vi "Trio - Disconnect.vi"(9 "TrioData In":T1 {"A Axis Parameters"."VPSPEED" format="%#_4g"; "A Axis Parameters"."AXISSTATUS" format="%#_4g"; "A Axis Parameters"."FE" format="%#_4g"; "A Axis Parameters"."MPOS" format="%#_4g"; "A Axis Parameters"."NTYPE" format="%#_4g"; "A Axis Parameters"."MTYPE" format="%#_4g"; "A Axis Parameters"."RS_LIMIT" format="%#_4g"; "A Axis Parameters"."FS_LIMIT" format="%#_4g"; "A Axis Parameters"."FH_IN" format="%#_4g"; "A Axis Parameters"."DATUM_IN" format="%#_4g"; "A Axis Parameters"."REV_IN" format="%#_4g"; "A Axis Parameters"."FWD_IN" format="%#_4g"; "A Axis Parameters"."REP_DIST" format="%#_4g"; "A Axis Parameters"."SERVO" format="%#_4g"; "A Axis Parameters"."DAC" format="%#_4g"; "A Axis Parameters"."FE_LIMIT" format="%#_4g"; "A Axis Parameters"."JOGSPEED" format="%#_4g"; "A Axis Parameters"."CREEP" format="%#_4g"; "A Axis Parameters"."DECEL" format="%#_4g"; "A Axis Parameters"."ACCEL" format="%#_4g"; "A Axis Parameters"."SPEED" format="%#_4g"; "A Axis Parameters"."UNITS" format="%#_4g"; "A Axis Parameters"."VFF_GAIN" format="%#_4g"; "A Axis Parameters"."0V_GAIN" format="%#_4g"; "A Axis Parameters"."D_GAIN" format="%#_4g"; "A Axis Parameters"."I_GAIN" format="%#_4g"; "A Axis Parameters"."P_GAIN" format="%#_4g"; "A Axis Parameters"."ATYPE" format="%#_4g"; "X Axis Parameters"."VPSPEED" format="%#_4g"; "X Axis Parameters"."AXISSTATUS" format="%#_4g"; "X Axis Parameters"."FE" format="%#_4g"; "X Axis Parameters"."MPOS" format="%#_4g"; "X Axis Parameters"."NTYPE" format="%#_4g"; "X Axis Parameters"."MTYPE" format="%#_4g"; "X Axis Parameters"."RS_LIMIT" format="%#_4g"; "X Axis Parameters"."FS_LIMIT" format="%#_4g"; "X Axis Parameters"."FH_IN" format="%#_4g"; "X Axis Parameters"."DATUM_IN" format="%#_4g"; "X Axis Parameters"."REV_IN" format="%#_4g"; "X Axis Parameters"."FWD_IN" format="%#_4g"; "X Axis Parameters"."REP_DIST" format="%#_4g"; "X Axis Parameters"."SERVO" format="%#_4g"; "X Axis Parameters"."DAC" format="%#_4g"; "X Axis Parameters"."FE_LIMIT" format="%#_4g"; "X Axis Parameters"."JOGSPEED" format="%#_4g"; "X Axis Parameters"."CREEP" format="%#_4g"; "X Axis Parameters"."DECEL" format="%#_4g"; "X Axis Parameters"."ACCEL" format="%#_4g"; "X Axis Parameters"."SPEED" format="%#_4g"; "X Axis Parameters"."UNITS" format="%#_4g"; "X Axis Parameters"."VFF_GAIN" format="%#_4g"; "X Axis Parameters"."0V_GAIN" format="%#_4g"; "X Axis Parameters"."D_GAIN" format="%#_4g"; "X Axis Parameters"."I_GAIN" format="%#_4g"; "X Axis Parameters"."P_GAIN" format="%#_4g"; "X Axis Parameters"."ATYPE" format="%#_4g"}, 10 "error in (no error)":errorcluster, 11 "Trio Reference In":refnum<k7>) -> (1 "TrioData Out":T1 {"A Axis Parameters"."VPSPEED" format="%#_4g"; "A Axis Parameters"."AXISSTATUS" format="%#_4g"; "A Axis Parameters"."FE" format="%#_4g"; "A Axis Parameters"."MPOS" format="%#_4g"; "A Axis Parameters"."NTYPE" format="%#_4g"; "A Axis Parameters"."MTYPE" format="%#_4g"; "A Axis Parameters"."RS_LIMIT" format="%#_4g"; "A Axis Parameters"."FS_LIMIT" format="%#_4g"; "A Axis Parameters"."FH_IN" format="%#_4g"; "A Axis Parameters"."DATUM_IN" format="%#_4g"; "A Axis Parameters"."REV_IN" format="%#_4g"; "A Axis Parameters"."FWD_IN" format="%#_4g"; "A Axis Parameters"."REP_DIST" format="%#_4g"; "A Axis Parameters"."SERVO" format="%#_4g"; "A Axis Parameters"."DAC" format="%#_4g"; "A Axis Parameters"."FE_LIMIT" format="%#_4g"; "A Axis Parameters"."JOGSPEED" format="%#_4g"; "A Axis Parameters"."CREEP" format="%#_4g"; "A Axis Parameters"."DECEL" format="%#_4g"; "A Axis Parameters"."ACCEL" format="%#_4g"; "A Axis Parameters"."SPEED" format="%#_4g"; "A Axis Parameters"."UNITS" format="%#_4g"; "A Axis Parameters"."VFF_GAIN" format="%#_4g"; "A Axis Parameters"."0V_GAIN" format="%#_4g"; "A Axis Parameters"."D_GAIN" format="%#_4g"; "A Axis Parameters"."I_GAIN" format="%#_4g"; "A Axis Parameters"."P_GAIN" format="%#_4g"; "A Axis Parameters"."ATYPE" format="%#_4g"; "X Axis Parameters"."VPSPEED" format="%#_4g"; "X Axis Parameters"."AXISSTATUS" format="%#_4g"; "X Axis Parameters"."FE" format="%#_4g"; "X Axis Parameters"."MPOS" format="%#_4g"; "X Axis Parameters"."NTYPE" format="%#_4g"; "X Axis Parameters"."MTYPE" format="%#_4g"; "X Axis Parameters"."RS_LIMIT" format="%#_4g"; "X Axis Parameters"."FS_LIMIT" format="%#_4g"; "X Axis Parameters"."FH_IN" format="%#_4g"; "X Axis Parameters"."DATUM_IN" format="%#_4g"; "X Axis Parameters"."REV_IN" format="%#_4g"; "X Axis Parameters"."FWD_IN" format="%#_4g"; "X Axis Parameters"."REP_DIST" format="%#_4g"; "X Axis Parameters"."SERVO" format="%#_4g"; "X Axis Parameters"."DAC" format="%#_4g"; "X Axis Parameters"."FE_LIMIT" format="%#_4g"; "X Axis Parameters"."JOGSPEED" format="%#_4g"; "X Axis Parameters"."CREEP" format="%#_4g"; "X Axis Parameters"."DECEL" format="%#_4g"; "X Axis Parameters"."ACCEL" format="%#_4g"; "X Axis Parameters"."SPEED" format="%#_4g"; "X Axis Parameters"."UNITS" format="%#_4g"; "X Axis Parameters"."VFF_GAIN" format="%#_4g"; "X Axis Parameters"."0V_GAIN" format="%#_4g"; "X Axis Parameters"."D_GAIN" format="%#_4g"; "X Axis Parameters"."I_GAIN" format="%#_4g"; "X Axis Parameters"."P_GAIN" format="%#_4g"; "X Axis Parameters"."ATYPE" format="%#_4g"}, 2 "error out":errorcluster, 3 "Trio Reference Out":refnum<k7>)   [LabVIEW 2020, in "TrioMotion Controller.lvlib"]
uses:
  TrioMotion Controller.lvlib
  TrioData.ctl
  Connection Type.ctl
  Axis Parameters.ctl
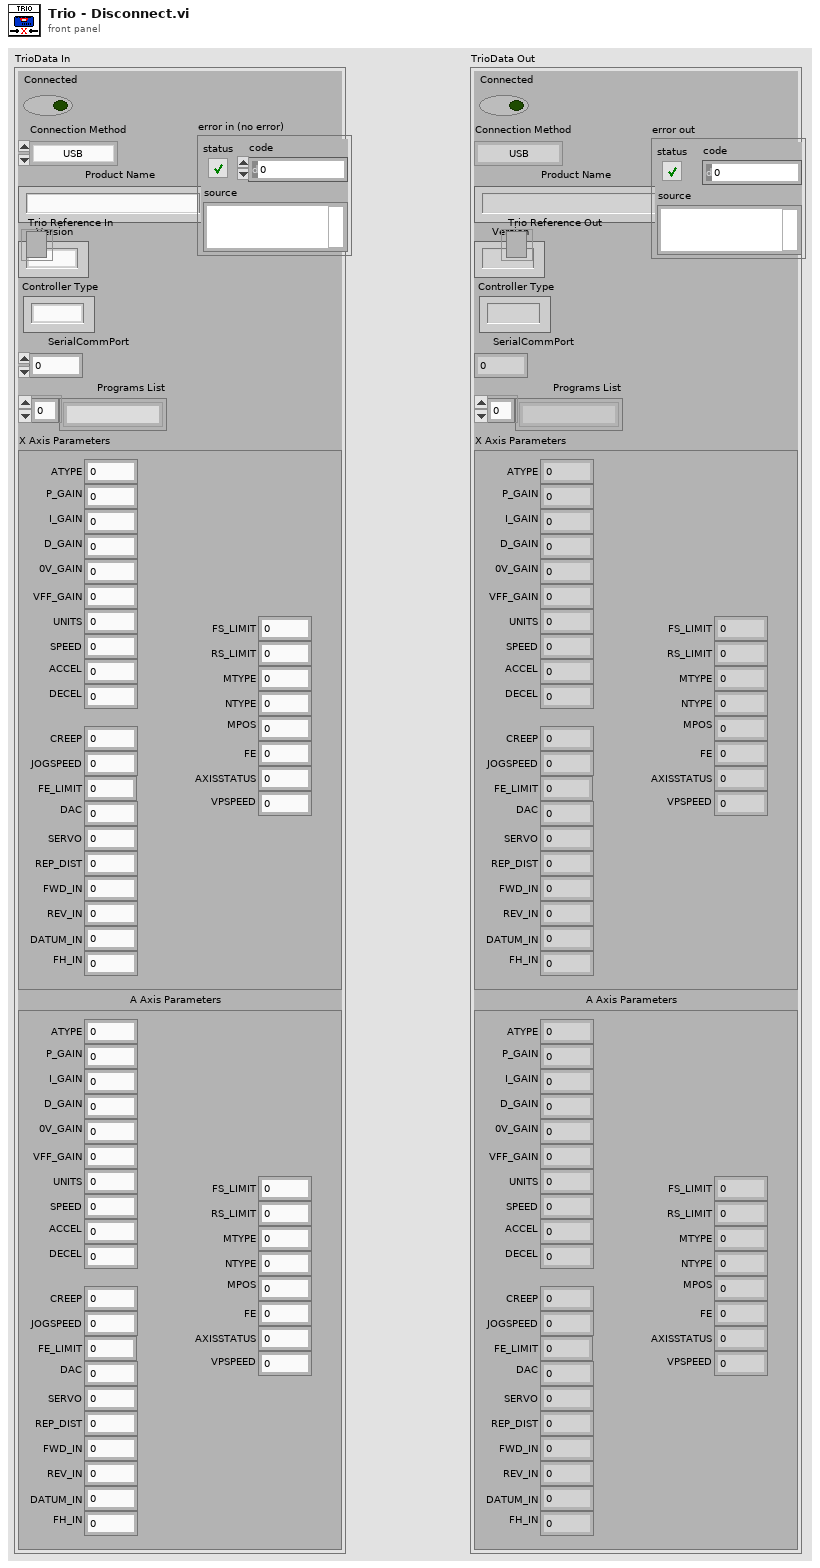
[diagram p1: front panel]
types:
  T1 = typedef "TrioMotion Controller.lvlib/TrioData.ctl" = cluster{"Connected":bool, "Connection Method":T2, "Product Name":string, " Version":string, "Controller Type":string, "SerialCommPort":fxp<+,3,3>, "Programs List":string[], "X Axis Parameters":T3, "A Axis Parameters":T3}
  T2 = typedef "TrioMotion Controller.lvlib/Connection Type.ctl" = enum16{"USB", "Serial", "Ethernet", "PCI", "Path", "No connection"}
  T3 = typedef "TrioMotion Controller.lvlib/Axis Parameters.ctl" = cluster{"ATYPE":dbl, "P_GAIN":dbl, "I_GAIN":dbl, "D_GAIN":dbl, "0V_GAIN":dbl, "VFF_GAIN":dbl, "UNITS":dbl, "SPEED":dbl, "ACCEL":dbl, "DECEL":dbl, "CREEP":dbl, "JOGSPEED":dbl, "FE_LIMIT":dbl, "DAC":dbl, "SERVO":dbl, "REP_DIST":dbl, "FWD_IN":dbl, "REV_IN":dbl, "DATUM_IN":dbl, "FH_IN":dbl, "FS_LIMIT":dbl, "RS_LIMIT":dbl, "MTYPE":dbl, "NTYPE":dbl, "MPOS":dbl, "FE":dbl, "AXISSTATUS":dbl, "VPSPEED":dbl}
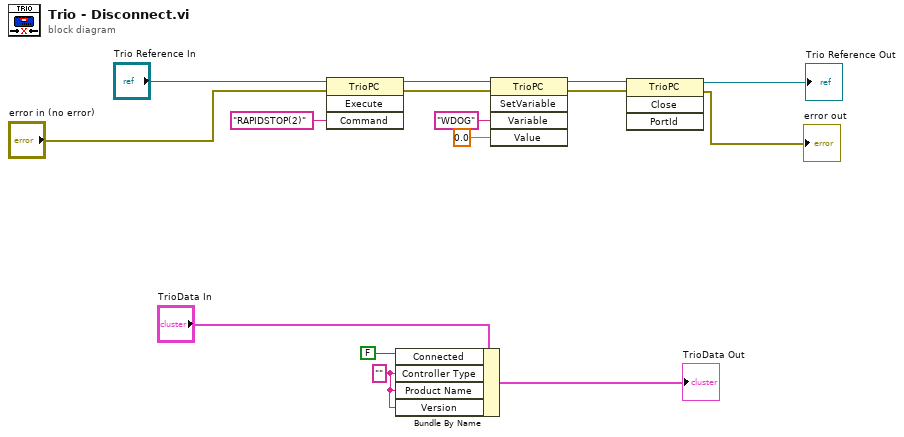
[diagram p0: block diagram]
diagram:
  w11 = "" ("Controller Type")
  n1 = invoke class="TrioPC" method="Execute"(reference="Trio Reference In", error in="error in (no error)", "Command"="RAPIDSTOP(2)") -> (reference out=w4:refnum<k7>, error out=w3:errorcluster)  [unwired: 1 in, 2 out]
  n2 = Bundle By Name(cluster="TrioData In", "Connected"=FALSE, "Controller Type"=w11, "Product Name"=w11, "Version"=w11) -> (→"TrioData Out":T1)
  n3 = invoke class="TrioPC" method="SetVariable"(reference=w4, error in=w3, "Variable"="WDOG", "Value"=0.0) -> (reference out=w2:refnum<k7>, error out=w1:errorcluster)  [unwired: 1 in, 3 out]
  n4 = invoke class="TrioPC" method="Close"(reference=w2, error in=w1) -> (reference out=→"Trio Reference Out":refnum<k7>, error out=→"error out":errorcluster)  [unwired: 2 in, 2 out]
